vi "updateConfig.vi"(11 "configuration file":path) -> ()   [LabVIEW 2012]
uses:
  variables/GlobalUI.vi
  <vilib>/Utility/config.llb/Write Key (Path).vi
  <vilib>/Utility/config.llb/Write Key (U32).vi
  <vilib>/Utility/config.llb/Write Key (Double).vi
  <vilib>/Utility/config.llb/Write Key (I32).vi
  <vilib>/Utility/config.llb/Write Key (String).vi
  <vilib>/Utility/config.llb/NI_LVConfig.lvlib
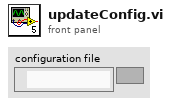
[diagram p1: front panel]
types:
  T1 = typedef "NI_LVConfig.lvlib/Config Data RefNum.ctl" = refnum<k1>
  T2 = typedef "Scan Parameters.ctl" = cluster{"x pixels":i32, "x voltage min":dbl, "x voltage max":dbl, "y voltage min":dbl, "y voltage max":dbl, "fill frac":dbl, "Zoom":dbl, "BiDi":bool, "scan rate (ms/line)":dbl}
  T3 = typedef "HWsettings.ctl" = cluster{"Galvo Channels":tag, "Detector Channels":tag, "Galvo Trigger":tag, "Shutter Lines":tag[], "Max Acquisition Rate":dbl, "Recommended Acquisition Rate":dbl, "Galvo Write Rate":dbl, "Max Timebase Frequency (Hz)":dbl, "MCC Shutter Lines":refnum<k21>[], "Detector Task":refnum<k21>, "Shutter Tasks":refnum<k21>[], "Galvo Task":refnum<k21>, "Digital Image Multiplier":dbl[]}
  T4 = typedef "Stage Parameters.ctl" = cluster{"Scan Mode":T5, "Start position mm":dbl, "End position mm":dbl, "Velocity um/sec (continuous)":dbl, "Step size microns (discrete)":dbl, "Frames to grab (grab)":i32}
  T5 = typedef "ScanMode.ctl" = enum16{"None", "Continuous", "Point Scan (CH3 cursor)", "Point Scan Move (CH3 cursor)", "Grab", "Grab Move Stage", "Grab Move Z-stage", "Cont. Move Z-stage", "Spec Move Stage", "Spec Move Cont", "Surf Calib"}
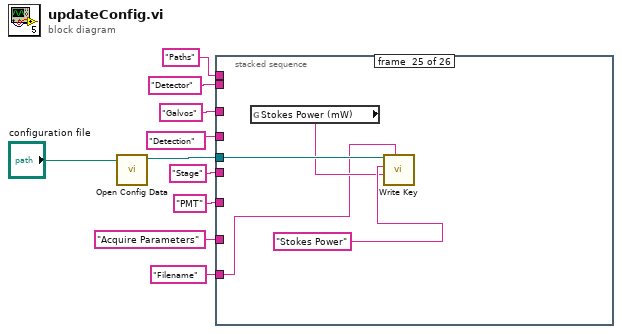
[diagram p0: block diagram]
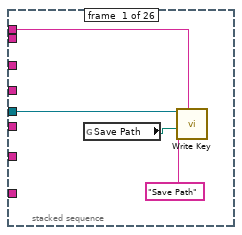
[diagram p2: hidden frame]
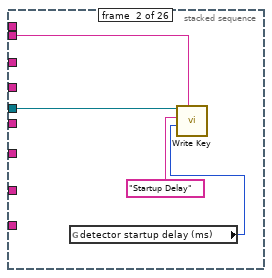
[diagram p3: hidden frame]
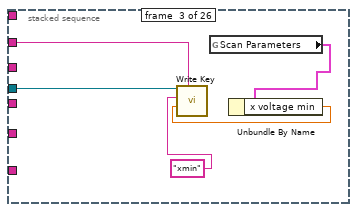
[diagram p4: hidden frame]
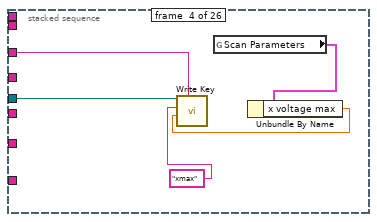
[diagram p5: hidden frame]
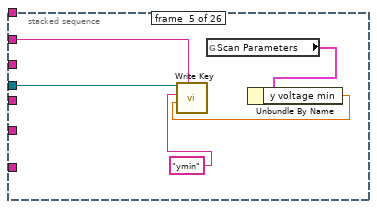
[diagram p6: hidden frame]
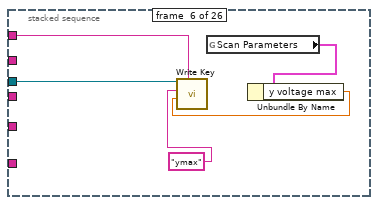
[diagram p7: hidden frame]
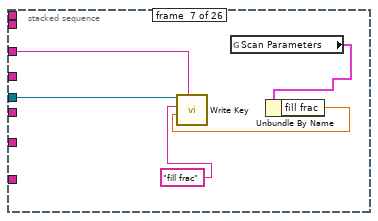
[diagram p8: hidden frame]
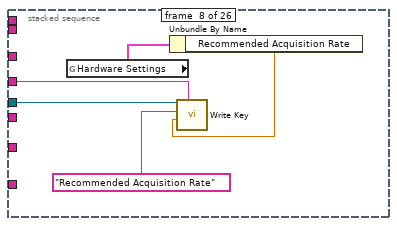
[diagram p9: hidden frame]
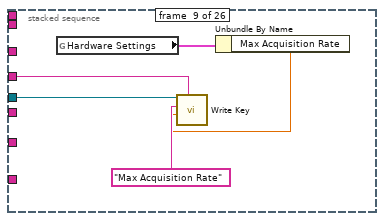
[diagram p10: hidden frame]
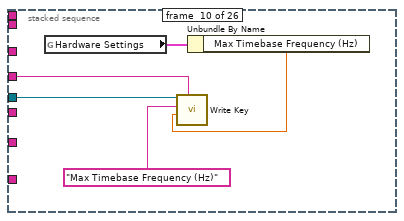
[diagram p11: hidden frame]
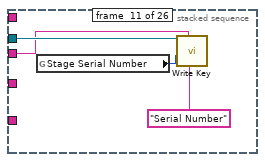
[diagram p12: hidden frame]
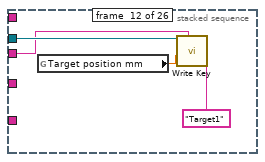
[diagram p13: hidden frame]
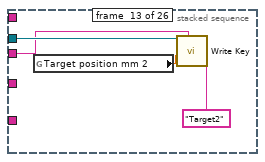
[diagram p14: hidden frame]
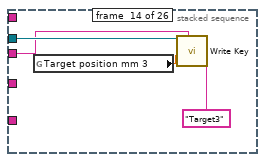
[diagram p15: hidden frame]
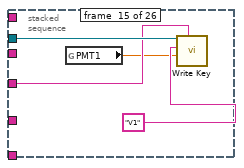
[diagram p16: hidden frame]
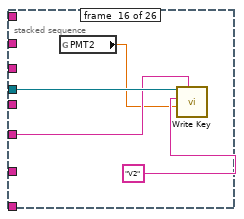
[diagram p17: hidden frame]
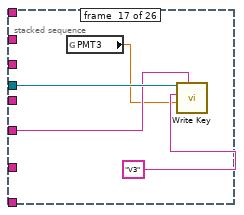
[diagram p18: hidden frame]
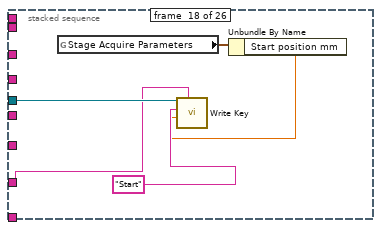
[diagram p19: hidden frame]
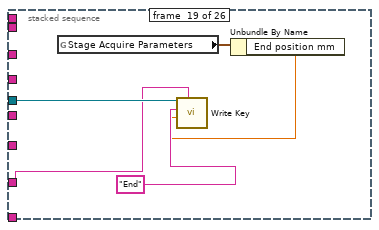
[diagram p20: hidden frame]
diagram:
  n1 = call <vilib>:"Open Config Data.vi"("configuration file path"="configuration file") -> ("refnum"=w3:T1)  [unwired: 8 in, 2 out]
  n2 = stacked-sequence {
    tunnel: w3 -> [w14 w18 w23 w28 w33 w38 w43 w48 w53 w58 w62 w66 w70 w74 w78 w82 w86 w91 w96 w101 w106 w111 w115 w119 w123 w124]
    tunnel: "Detection" ("section") -> [_ _ _ _ _ _ _ w46 w51 w56 _ _ _ _ _ _ _ _ _ _ _ _ _ _ _ _]
    tunnel: "Galvos" ("section") -> [_ _ w22 w27 w32 w37 w42 _ _ _ _ _ _ _ _ _ _ _ _ _ _ _ _ _ _ _]
    tunnel: "Detector" ("section") -> [_ w16 _ _ _ _ _ _ _ _ _ _ _ _ _ _ _ _ _ _ _ _ _ _ _ _]
    tunnel: "Paths" ("section") -> [w12 _ _ _ _ _ _ _ _ _ _ _ _ _ _ _ _ _ _ _ _ _ _ _ _ _]
    tunnel: "Stage" ("section") -> [_ _ _ _ _ _ _ _ _ _ w60 w64 w68 w72 _ _ _ _ _ _ _ _ _ _ _ _]
    tunnel: "PMT" ("section") -> [_ _ _ _ _ _ _ _ _ _ _ _ _ _ w76 w80 w84 _ _ _ _ _ _ _ _ _]
    tunnel: "Acquire Parameters" ("section") -> [_ _ _ _ _ _ _ _ _ _ _ _ _ _ _ _ _ w88 w93 w98 w103 w108 _ _ _ _]
    tunnel: "Filename" ("section") -> [_ _ _ _ _ _ _ _ _ _ _ _ _ _ _ _ _ _ _ _ _ _ w112 w116 w120 _]
    frame #0 {
      n3 = global read "GlobalUI.vi" "Save Path"() -> (w11:path)
      n4 = call-poly <vilib>:"Write Key.vi"("section"=w12, "value"=w11, "key"="Save Path", "refnum"=w14) -> ()  [unwired: 5 in, 3 out]
    }
    frame #1 {
      n5 = global read "GlobalUI.vi" "detector startup delay (ms)"() -> (w15:u32)
      n6 = call-poly <vilib>:"Write Key.vi"("section"=w16, "value"=w15, "key"="Startup Delay", "refnum"=w18) -> ()  [unwired: 5 in, 3 out]
    }
    frame #2 {
      n7 = global read "GlobalUI.vi" "Scan Parameters"() -> (w19:T2)
      n8 = Unbundle By Name(w19) -> ("x voltage min"=w21:dbl)
      n9 = call-poly <vilib>:"Write Key.vi"("section"=w22, "value"=w21, "key"="xmin", "refnum"=w23) -> ()  [unwired: 5 in, 3 out]
    }
    frame #3 {
      n10 = global read "GlobalUI.vi" "Scan Parameters"() -> (w24:T2)
      n11 = Unbundle By Name(w24) -> ("x voltage max"=w25:dbl)
      n12 = call-poly <vilib>:"Write Key.vi"("section"=w27, "value"=w25, "key"="xmax", "refnum"=w28) -> ()  [unwired: 5 in, 3 out]
    }
    frame #4 {
      n13 = global read "GlobalUI.vi" "Scan Parameters"() -> (w29:T2)
      n14 = Unbundle By Name(w29) -> ("y voltage min"=w30:dbl)
      n15 = call-poly <vilib>:"Write Key.vi"("section"=w32, "value"=w30, "key"="ymin", "refnum"=w33) -> ()  [unwired: 5 in, 3 out]
    }
    frame #5 {
      n16 = global read "GlobalUI.vi" "Scan Parameters"() -> (w34:T2)
      n17 = Unbundle By Name(w34) -> ("y voltage max"=w35:dbl)
      n18 = call-poly <vilib>:"Write Key.vi"("section"=w37, "value"=w35, "key"="ymax", "refnum"=w38) -> ()  [unwired: 5 in, 3 out]
    }
    frame #6 {
      n19 = global read "GlobalUI.vi" "Scan Parameters"() -> (w39:T2)
      n20 = Unbundle By Name(w39) -> ("fill frac"=w40:dbl)
      n21 = call-poly <vilib>:"Write Key.vi"("section"=w42, "value"=w40, "key"="fill frac", "refnum"=w43) -> ()  [unwired: 5 in, 3 out]
    }
    frame #7 {
      n22 = global read "GlobalUI.vi" "Hardware Settings"() -> (w44:T3)
      n23 = Unbundle By Name(w44) -> ("Recommended Acquisition Rate"=w45:dbl)
      n24 = call-poly <vilib>:"Write Key.vi"("section"=w46, "value"=w45, "key"="Recommended Acquisition Rate", "refnum"=w48) -> ()  [unwired: 5 in, 3 out]
    }
    frame #8 {
      n25 = global read "GlobalUI.vi" "Hardware Settings"() -> (w49:T3)
      n26 = Unbundle By Name(w49) -> ("Max Acquisition Rate"=w50:dbl)
      n27 = call-poly <vilib>:"Write Key.vi"("section"=w51, "value"=w50, "key"="Max Acquisition Rate", "refnum"=w53) -> ()  [unwired: 5 in, 3 out]
    }
    frame #9 {
      n28 = global read "GlobalUI.vi" "Hardware Settings"() -> (w54:T3)
      n29 = Unbundle By Name(w54) -> ("Max Timebase Frequency (Hz)"=w55:dbl)
      n30 = call-poly <vilib>:"Write Key.vi"("section"=w56, "value"=w55, "key"="Max Timebase Frequency (Hz)", "refnum"=w58) -> ()  [unwired: 5 in, 3 out]
    }
    frame #10 {
      n31 = global read "GlobalUI.vi" "Stage Serial Number"() -> (w59:i32)
      n32 = call-poly <vilib>:"Write Key.vi"("section"=w60, "value"=w59, "key"="Serial Number", "refnum"=w62) -> ()  [unwired: 5 in, 3 out]
    }
    frame #11 {
      n33 = global read "GlobalUI.vi" "Target position mm"() -> (w63:dbl)
      n34 = call-poly <vilib>:"Write Key.vi"("section"=w64, "value"=w63, "key"="Target1", "refnum"=w66) -> ()  [unwired: 5 in, 3 out]
    }
    frame #12 {
      n35 = global read "GlobalUI.vi" "Target position mm 2"() -> (w67:dbl)
      n36 = call-poly <vilib>:"Write Key.vi"("section"=w68, "value"=w67, "key"="Target2", "refnum"=w70) -> ()  [unwired: 5 in, 3 out]
    }
    frame #13 {
      n37 = global read "GlobalUI.vi" "Target position mm 3"() -> (w71:dbl)
      n38 = call-poly <vilib>:"Write Key.vi"("section"=w72, "value"=w71, "key"="Target3", "refnum"=w74) -> ()  [unwired: 5 in, 3 out]
    }
    frame #14 {
      n39 = global read "GlobalUI.vi" "PMT1"() -> (w75:dbl)
      n40 = call-poly <vilib>:"Write Key.vi"("section"=w76, "value"=w75, "key"="V1", "refnum"=w78) -> ()  [unwired: 5 in, 3 out]
    }
    frame #15 {
      n41 = global read "GlobalUI.vi" "PMT2"() -> (w79:dbl)
      n42 = call-poly <vilib>:"Write Key.vi"("section"=w80, "value"=w79, "key"="V2", "refnum"=w82) -> ()  [unwired: 5 in, 3 out]
    }
    frame #16 {
      n43 = global read "GlobalUI.vi" "PMT3"() -> (w83:dbl)
      n44 = call-poly <vilib>:"Write Key.vi"("section"=w84, "value"=w83, "key"="V3", "refnum"=w86) -> ()  [unwired: 5 in, 3 out]
    }
    frame #17 {
      n45 = global read "GlobalUI.vi" "Stage Acquire Parameters"() -> (w89:T4)
      n46 = Unbundle By Name(w89) -> ("Start position mm"=w87:dbl)
      n47 = call-poly <vilib>:"Write Key.vi"("section"=w88, "value"=w87, "key"="Start", "refnum"=w91) -> ()  [unwired: 5 in, 3 out]
    }
    frame #18 {
      n48 = global read "GlobalUI.vi" "Stage Acquire Parameters"() -> (w94:T4)
      n49 = Unbundle By Name(w94) -> ("End position mm"=w92:dbl)
      n50 = call-poly <vilib>:"Write Key.vi"("section"=w93, "value"=w92, "key"="End", "refnum"=w96) -> ()  [unwired: 5 in, 3 out]
    }
    frame #19 {
      n51 = global read "GlobalUI.vi" "Stage Acquire Parameters"() -> (w99:T4)
      n52 = Unbundle By Name(w99) -> ("Velocity um/sec (continuous)"=w97:dbl)
      n53 = call-poly <vilib>:"Write Key.vi"("section"=w98, "value"=w97, "key"="Velocity", "refnum"=w101) -> ()  [unwired: 5 in, 3 out]
    }
    frame #20 {
      n54 = global read "GlobalUI.vi" "Stage Acquire Parameters"() -> (w104:T4)
      n55 = Unbundle By Name(w104) -> ("Step size microns (discrete)"=w102:dbl)
      n56 = call-poly <vilib>:"Write Key.vi"("section"=w103, "value"=w102, "key"="Step size", "refnum"=w106) -> ()  [unwired: 5 in, 3 out]
    }
    frame #21 {
      n57 = global read "GlobalUI.vi" "Stage Acquire Parameters"() -> (w109:T4)
      n58 = Unbundle By Name(w109) -> ("Frames to grab (grab)"=w107:i32)
      n59 = call-poly <vilib>:"Write Key.vi"("section"=w108, "value"=w107, "key"="Frames to grab", "refnum"=w111) -> ()  [unwired: 5 in, 3 out]
    }
    frame #22 {
      n60 = global read "GlobalUI.vi" "Sample Description"() -> (w113:string)
      n61 = call-poly <vilib>:"Write Key.vi"("section"=w112, "value"=w113, "key"="Sample Description", "refnum"=w115) -> ()  [unwired: 5 in, 3 out]
    }
    frame #23 {
      n62 = global read "GlobalUI.vi" "Pump Power (mW)"() -> (w117:string)
      n63 = call-poly <vilib>:"Write Key.vi"("section"=w116, "value"=w117, "key"="Pump Power", "refnum"=w119) -> ()  [unwired: 5 in, 3 out]
    }
    frame #24 {
      n64 = global read "GlobalUI.vi" "Stokes Power (mW)"() -> (w121:string)
      n65 = call-poly <vilib>:"Write Key.vi"("section"=w120, "value"=w121, "key"="Stokes Power", "refnum"=w123) -> ()  [unwired: 5 in, 3 out]
    }
    frame #25 {
      n66 = call <vilib>:"Close Config Data.vi"("refnum"=w124) -> ()  [unwired: 9 in, 2 out]
    }
  }
